vi "AuMT8852B Connection Packets.vi"(5 "Packet Types (all used)":T1, 7 "Set/Get (Set)":enum16{"Set", "Get"}(ring), 8 "error in (no error)":errorcluster, 11 "VISA session":refnum<visa-resource-name>) -> (0 "error out":errorcluster, 2 "error code":i32, 3 "VISA session out":refnum<visa-resource-name>, 4 "Packet Types":T1)   [LabVIEW 2017]
doc: "Anritsu MT8852B Bluetooth Tester\n\nSpecifies which packet types the Link Manager shall use for the ACL connection.\n\nINPUTS\nSet/Get - whether the values are being written to or read from the instrument.\nPacket Types - the status of packet types available for the ACL connection.\n\nOUTPUTS\nPacket Types out - the current status of the range of packet types available for the ACL connection."
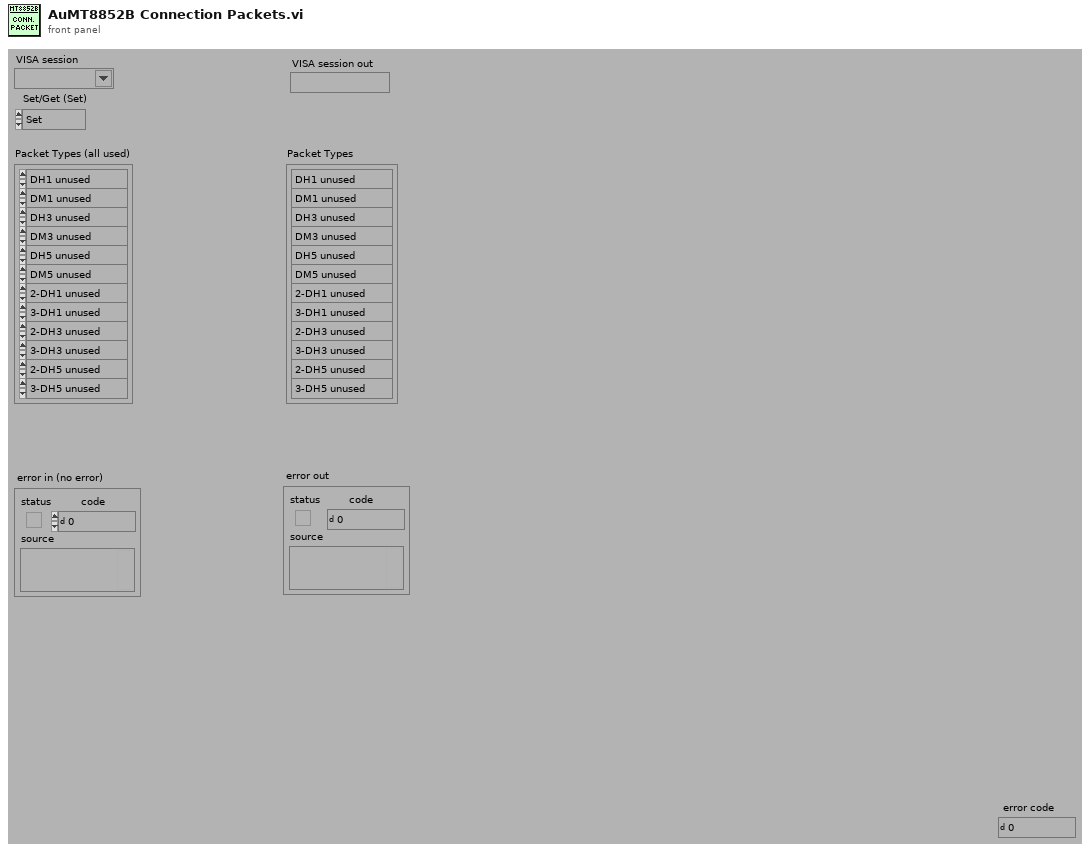
[diagram p1: front panel]
types:
  T1 = cluster{"DH1":enum16{"DH1 unused", "DH1 used"}, "DM1":enum16{"DM1 unused", "DM1 used"}, "DH3":enum16{"DH3 unused", "DH3 used"}, "DM3":enum16{"DM3 unused", "DM3 used"}, "DH5":enum16{"DH5 unused", "DH5 used"}, "DM5":enum16{"DM5 unused", "DM5 used"}, "2-DH1":enum16{"2-DH1 unused", "2-DH1 used"}, "3-DH1":enum16{"3-DH1 unused", "3-DH1 used"}, "2-DH3":enum16{"2-DH3 unused", "2-DH3 used"}, "3-DH3":enum16{"3-DH3 unused", "3-DH3 used"}, "2-DH5":enum16{"2-DH5 unused", "2-DH5 used"}, "3-DH5":enum16{"3-DH5 unused", "3-DH5 used"}}
  T2 = enum16{"Simulate", "Range check", "Cache", "Query instrument status"}
  T3 = cluster{"[0]":i16, "[1]":i16, "[2]":i16, "[3]":i16, "[4]":i16, "[5]":i16, "[6]":i16, "[7]":i16, "[8]":i16, "[9]":i16, "[10]":i16, "[11]":i16}
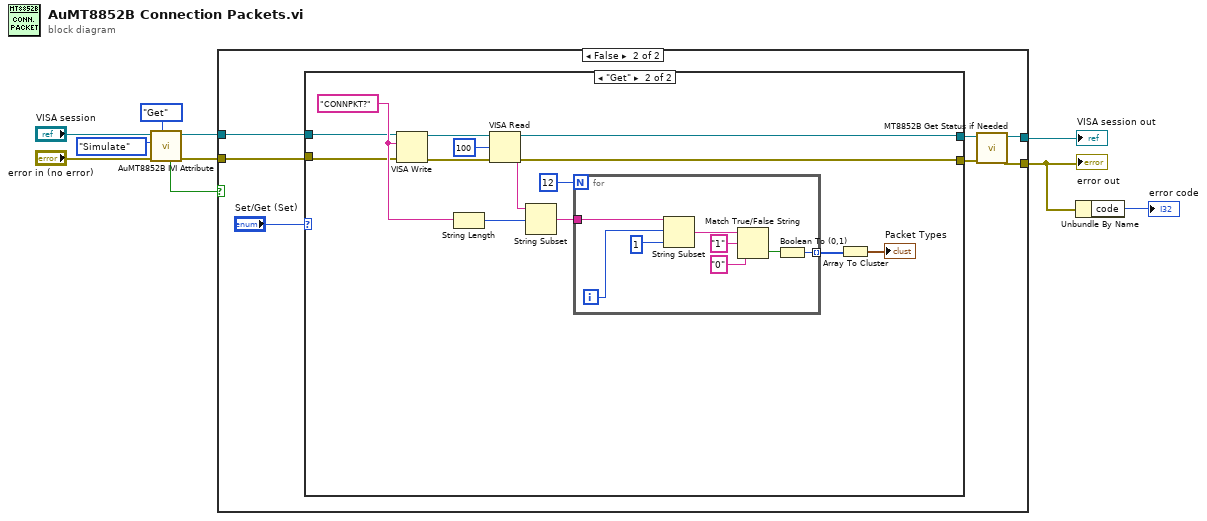
[diagram p0: block diagram]
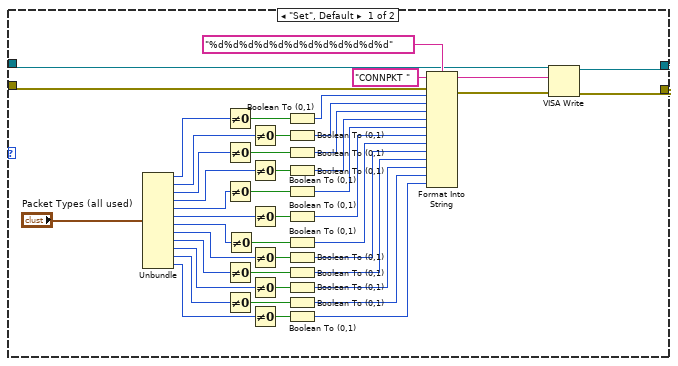
[diagram p3: hidden frame]
diagram:
  n1 = call <instrlib>:"AuMT8852B IVI Attribute.vi"("Set/Get (Set)"=enum16{"Set", "Get"}."Get", "error in (no error)"="error in (no error)", "Flag (Simulate)"=T2."Simulate", "VISA session"="VISA session") -> ("error out"=w4:errorcluster, "VISA session out"=w6:refnum<visa-resource-name>, "Value out"=w5:bool)  [unwired: 5 in]
  n2 = case shown="False" w5 {
    tunnel: w6 -> [w12 w17]
    tunnel: w4 -> [w11 w18]
    tunnel: [w11 w15] -> w1
    tunnel: [w12 w14] -> w3
    frame True {
    }
    frame False {
      n3 = case shown="\"Get\"" "Set/Get (Set)" {
        tunnel: w18 -> [w25 w72]
        tunnel: [w24 w68] -> w16
        tunnel: [w22 w69] -> w13
        tunnel: w17 -> [w21 w73]
        frame "Set", Default {
          n4 = Unbundle("Packet Types (all used)") -> ("DH1"=w27:enum16{"DH1 unused", "DH1 used"}, "DM1"=w28:enum16{"DM1 unused", "DM1 used"}, "DH3"=w29:enum16{"DH3 unused", "DH3 used"}, "DM3"=w30:enum16{"DM3 unused", "DM3 used"}, "DH5"=w32:enum16{"DH5 unused", "DH5 used"}, "DM5"=w31:enum16{"DM5 unused", "DM5 used"}, "2-DH1"=w33:enum16{"2-DH1 unused", "2-DH1 used"}, "3-DH1"=w34:enum16{"3-DH1 unused", "3-DH1 used"}, "2-DH3"=w35:enum16{"2-DH3 unused", "2-DH3 used"}, "3-DH3"=w36:enum16{"3-DH3 unused", "3-DH3 used"}, "2-DH5"=w37:enum16{"2-DH5 unused", "2-DH5 used"}, "3-DH5"=w61:enum16{"3-DH5 unused", "3-DH5 used"})
          n5 = Not Equal To 0?(x=w27) -> (x != 0?=w38:bool)
          n6 = Not Equal To 0?(x=w29) -> (x != 0?=w40:bool)
          n7 = Not Equal To 0?(x=w32) -> (x != 0?=w62:bool)
          n8 = Not Equal To 0?(x=w35) -> (x != 0?=w45:bool)
          n9 = Not Equal To 0?(x=w37) -> (x != 0?=w47:bool)
          n10 = Not Equal To 0?(x=w33) -> (x != 0?=w43:bool)
          n11 = Not Equal To 0?(x=w28) -> (x != 0?=w39:bool)
          n12 = Not Equal To 0?(x=w30) -> (x != 0?=w41:bool)
          n13 = Not Equal To 0?(x=w31) -> (x != 0?=w42:bool)
          n14 = Not Equal To 0?(x=w34) -> (x != 0?=w44:bool)
          n15 = Not Equal To 0?(x=w36) -> (x != 0?=w46:bool)
          n16 = Not Equal To 0?(x=w61) -> (x != 0?=w48:bool)
          n17 = Boolean To (0,1)(Boolean=w38) -> (0, 1=w49:i16)
          n18 = Boolean To (0,1)(Boolean=w39) -> (0, 1=w50:i16)
          n19 = Boolean To (0,1)(Boolean=w40) -> (0, 1=w51:i16)
          n20 = Boolean To (0,1)(Boolean=w41) -> (0, 1=w63:i16)
          n21 = Boolean To (0,1)(Boolean=w62) -> (0, 1=w52:i16)
          n22 = Boolean To (0,1)(Boolean=w42) -> (0, 1=w53:i16)
          n23 = Boolean To (0,1)(Boolean=w43) -> (0, 1=w54:i16)
          n24 = Boolean To (0,1)(Boolean=w44) -> (0, 1=w55:i16)
          n25 = Boolean To (0,1)(Boolean=w45) -> (0, 1=w56:i16)
          n26 = Boolean To (0,1)(Boolean=w46) -> (0, 1=w57:i16)
          n27 = Boolean To (0,1)(Boolean=w47) -> (0, 1=w58:i16)
          n28 = Boolean To (0,1)(Boolean=w48) -> (0, 1=w59:i16)
          n29 = Format Into String(format string="%d%d%d%d%d%d%d%d%d%d%d%d", initial string="CONNPKT ", error in=w25, w49, w50, w51, w63, w52, w53, w54, w55, w56, w57, w58, w59) -> (resulting string=w60:string, error out=w23:errorcluster)
          n30 = VISA Write(VISA resource name=w21, write buffer=w60, error in (no error)=w23) -> (VISA resource name out=w22:refnum<visa-resource-name>, error out=w24:errorcluster)  [unwired: 1 out]
        }
        frame "Get" {
          w74 = "CONNPKT?"
          n31 = VISA Write(VISA resource name=w73, write buffer=w74, error in (no error)=w72) -> (VISA resource name out=w76:refnum<visa-resource-name>, error out=w78:errorcluster)  [unwired: 1 out]
          n32 = String Length(string=w74) -> (length=w71:i32)
          n33 = VISA Read(VISA resource name=w76, byte count=u32 100 ("byte count (0)"), error in (no error)=w78) -> (VISA resource name out=w69:refnum<visa-resource-name>, read buffer=w75:string, error out=w68:errorcluster)  [unwired: 1 out]
          n34 = String Subset(string=w75, offset (0)=w71) -> (substring=w66:string)  [unwired: 1 in]
          n35 = for {
            N: 12 ("offset (0)") -> [_]
            tunnel: w66 -> [w86]
            tunnel: [w79] -> w67 mode=indexing
            i -> [w85]
            n36 = String Subset(string=w86, offset (0)=w85, length (rest)=1 ("length (rest)")) -> (substring=w81:string)
            n37 = Match True/False String(2:"0" ("false string"), 3:"1" ("true string"), 4:w81) -> (0:w80:bool)  [unwired: 1 out]
            n38 = Boolean To (0,1)(Boolean=w80) -> (0, 1=w79:i16)
          }
          n39 = Array To Cluster(array=w67) -> (cluster=→"Packet Types":T3)
        }
      }
      n40 = call <instrlib>:"MT8852B Get Status if Needed.vi"("error in (no error)"=w16, "VISA session"=w13) -> ("error out"=w15:errorcluster, "VISA session out"=w14:refnum<visa-resource-name>)  [unwired: 8 in]
    }
  }
  "error out" <- w1
  "VISA session out" <- w3
  n41 = Unbundle By Name(w1) -> ("code"=→"error code":i32)
